vi "LEP_RV_PrepareBuild.vi"(5 "Rebuild":bool, 11 "error in (no error)":errorcluster) -> (0 "error string":string, 1 "Node ID List":i32[](array[numeric]), 2 "Active File Count":i32, 3 "TopLevelVI":path, 4 "UV License OK":bool, 6 "Config":T1={"Enable debugging"=FALSE, "Debug Options"=0, "Use stack variables"=FALSE, "Generate serial only"=FALSE, "Generate guard code"=TRUE, "Generate Integer Only"=TRUE, "Generate C Function Calls"=TRUE, "ExpressionFolding"=FALSE, "Constant Allocation"=0, "Constant Deallocation"=0, "Build Specification ID"="", "Preprocessor symbols (define)"="", "Compiler Flags"="", "Linker Flags"="", "Mode"=1, "Optimization"=2, "Optimize for time"=FALSE, "Enable cross-module optimization"=FALSE, "Include paths"=[], "Optimize heap size"=TRUE, "Use MicroLib"=FALSE, "Debug Mode"=2, "Enable profile information"=FALSE, "Host name"="board", "Use DHCP"=TRUE, "IP address"="0.0.0.0", "Subnet mask"="", "Gateway"="0.0.0.0", "Primary DNS"="0.0.0.0", "Secondary DNS"="0.0.0.0", "MAC in target memory"=TRUE, "MAC address"="", "Console output"=1, "Target serial port"=1} {"Constant Deallocation" items=["Out of Scope", "VI End", "Application End"]; "Constant Allocation" items=["First Use", "Containing Loop", "VI Initialization", "Application Initialization"]; "Target serial port" items=["0", "1", "2", "3"]; "Console output" items=["Processor status window", "Serial port"]; "Optimization" items=["Level 0 (-O0)", "Level 1 (-O1)", "Level 2 (-O2)", "Level 3 (-O3)"]; "Mode" items=["ARM-Mode", "Thumb-Mode"]; "Debug Options" items=["Use ULINK Debugger", "Use Simulator"]; "Debug Mode" items=["Instrumented (serial port)", "Instrumented (TCP/IP)", "Non-instrumented (JTAG/USB)"]}, 8 "Build Path":path, 10 "Target Name":string, 12 "Message List":string[][](array[string]), 13 "Error Indicator":bool[](array[boolean]), 14 "UV Project File":path, 15 "error out":errorcluster)   [LabVIEW 2011]
doc: "Loads project configuration information, creates the build folder, prepares the source files, builds, and links the embedded application."
uses:
  LEP_RV_Config.ctl
panel:
  out "Executable file":path
  in  "Build Path":path
  in  "Config":T1={"Enable debugging"=FALSE, "Debug Options"=0, "Use stack variables"=FALSE, "Generate serial only"=FALSE, "Generate guard code"=FALSE, "Generate Integer Only"=FALSE, "Generate C Function Calls"=TRUE, "ExpressionFolding"=TRUE, "Constant Allocation"=0, "Constant Deallocation"=0, "Build Specification ID"="", "Preprocessor symbols (define)"="", "Compiler Flags"="", "Linker Flags"="", "Mode"=1, "Optimization"=2, "Optimize for time"=FALSE, "Enable cross-module optimization"=FALSE, "Include paths"=[], "Optimize heap size"=TRUE, "Use MicroLib"=FALSE, "Debug Mode"=2, "Enable profile information"=FALSE, "Host name"="board", "Use DHCP"=TRUE, "IP address"="0.0.0.0", "Subnet mask"="", "Gateway"="0.0.0.0", "Primary DNS"="0.0.0.0", "Secondary DNS"="0.0.0.0", "MAC in target memory"=TRUE, "MAC address"="", "Console output"=1, "Target serial port"=1} {"Constant Deallocation" items=["Out of Scope", "VI End", "Application End"]; "Constant Allocation" items=["First Use", "Containing Loop", "VI Initialization", "Application Initialization"]; "Target serial port" items=["0", "1", "2", "3"]; "Console output" items=["Processor status window", "Serial port"]; "Optimization" items=["Level 0 (-O0)", "Level 1 (-O1)", "Level 2 (-O2)", "Level 3 (-O3)"]; "Mode" items=["ARM-Mode", "Thumb-Mode"]; "Debug Options" items=["Use ULINK Debugger", "Use Simulator"]; "Debug Mode" items=["Instrumented (serial port)", "Instrumented (TCP/IP)", "Non-instrumented (JTAG/USB)"]}
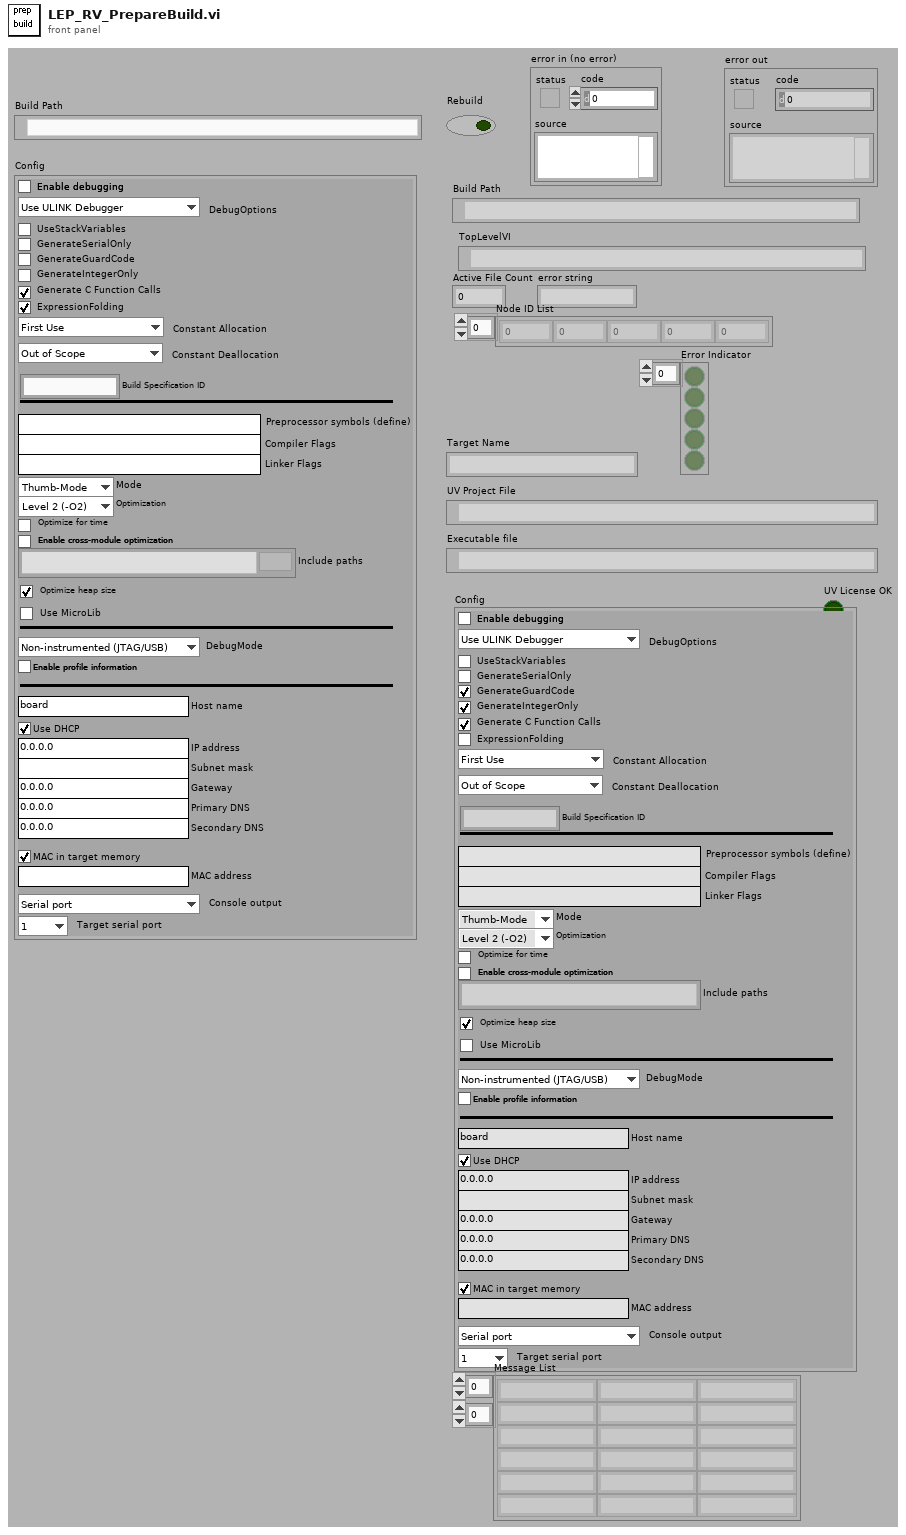
[diagram p1: front panel]
types:
  T1 = typedef "LEP_RV_Config.ctl" = cluster{"Enable debugging":bool, "Debug Options":u16, "Use stack variables":bool, "Generate serial only":bool, "Generate guard code":bool, "Generate Integer Only":bool, "Generate C Function Calls":bool, "ExpressionFolding":bool, "Constant Allocation":u16, "Constant Deallocation":u16, "Build Specification ID":string, "Preprocessor symbols (define)":string, "Compiler Flags":string, "Linker Flags":string, "Mode":u16, "Optimization":u16, "Optimize for time":bool, "Enable cross-module optimization":bool, "Include paths":path[], "Optimize heap size":bool, "Use MicroLib":bool, "Debug Mode":u16, "Enable profile information":bool, "Host name":string, "Use DHCP":bool, "IP address":string, "Subnet mask":string, "Gateway":string, "Primary DNS":string, "Secondary DNS":string, "MAC in target memory":bool, "MAC address":string, "Console output":u16, "Target serial port":u16}
  T2 = enum16{"NoErr", "TopLevelVIErr", "EmptyTopLevelVIPath", "CGenErr", "CpySuppFilesErr", "ProjectInfoErr", "NoTopLevelVIErr", "CreateBuildFolderErr", "EmptyBuildFolderErr", "LoadConfigErr", "BildToolsErr", "CompileErr", "LinkError", "DebugInfoErr", "NotFoundErr", "AccessErr", "ExecErr", "UnknownErr", "ISRErr"}
  T3 = enum16{"LoadProjectInfo", "LoadConfig", "SetupBuildFolder", "CopySupportFiles", "CGen", "CreateUVProject", "ConfigureUVproject", "BuildwithUV", "GenerateDebugDatabase", "ShowUserMessage", "Done", "Error"}
  T4 = enum16{"Normal", "Minimized", "Maximized", "Hidden", "Locked"}
  T5 = enum16{"NoErr", "TopLevelVIErr", "EmptyTopLevelVIPath", "CGenErr", "CpySuppFilesErr", "ProjectInfoErr", "NoTopLevelVIErr", "CreateBuildFolderErr", "EmptyBuildFolderErr", "LoadConfigErr", "BildToolsErr", "CompileErr", "LinkError", "DebugInfoErr", "NotFoundErr", "AccessErr", "ExecErr", "UnknownErr"}
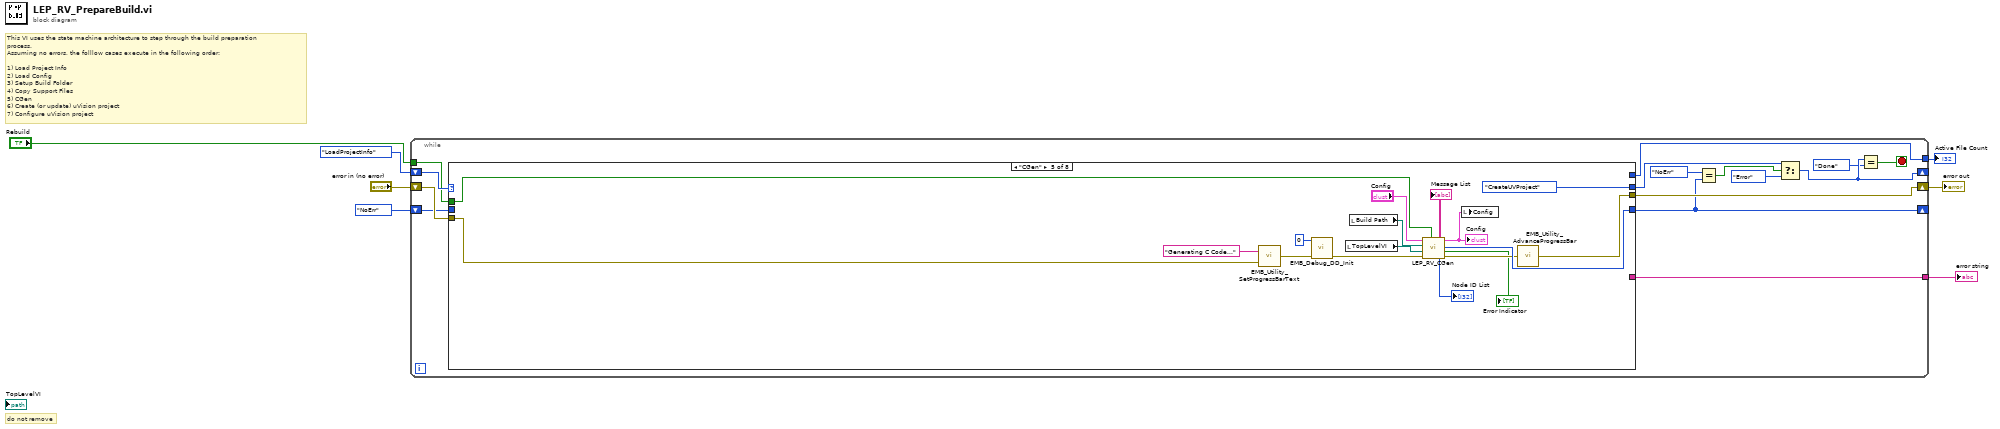
[diagram p0: block diagram]
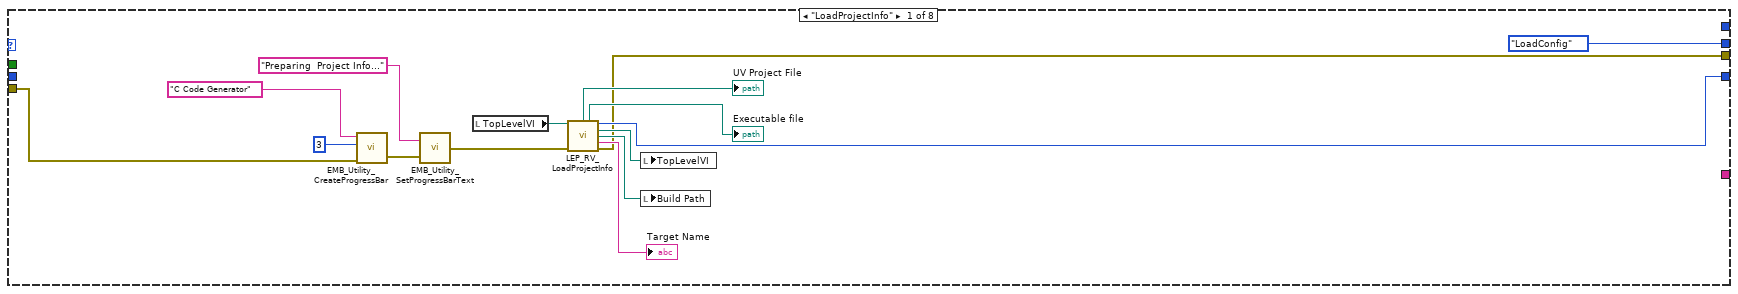
[diagram p2: hidden frame]
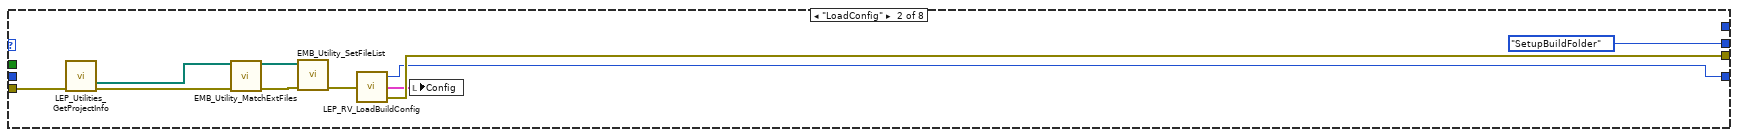
[diagram p3: hidden frame]
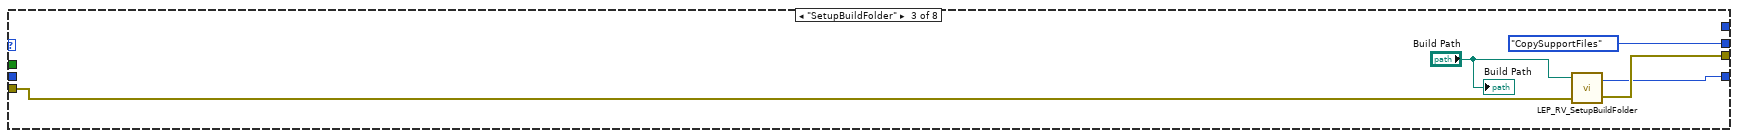
[diagram p4: hidden frame]
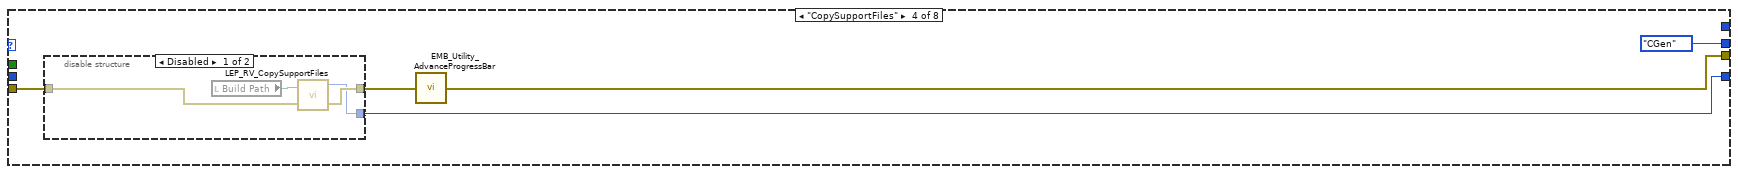
[diagram p5: hidden frame]
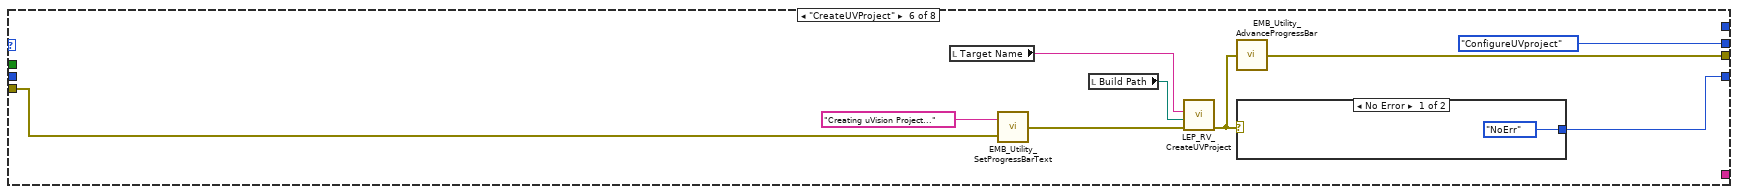
[diagram p7: hidden frame]
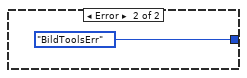
[diagram p8: hidden frame]
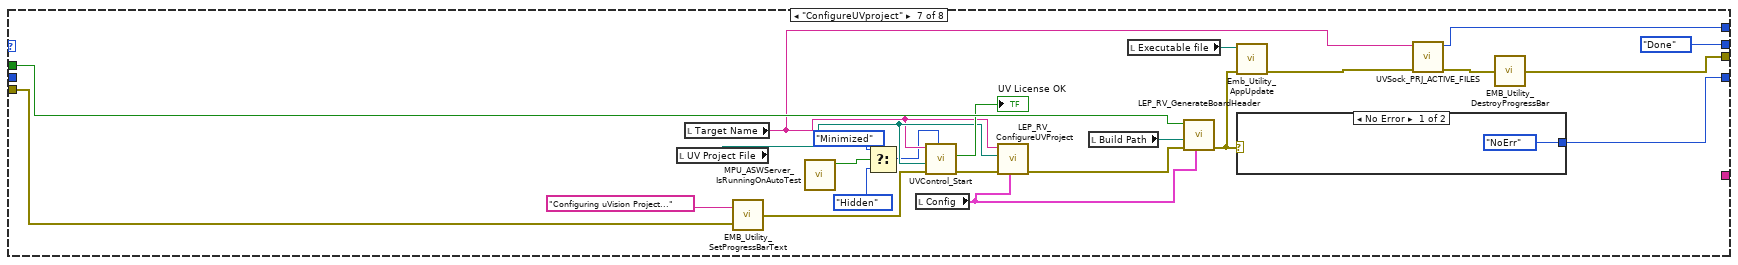
[diagram p9: hidden frame]
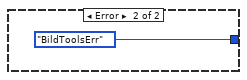
[diagram p10: hidden frame]
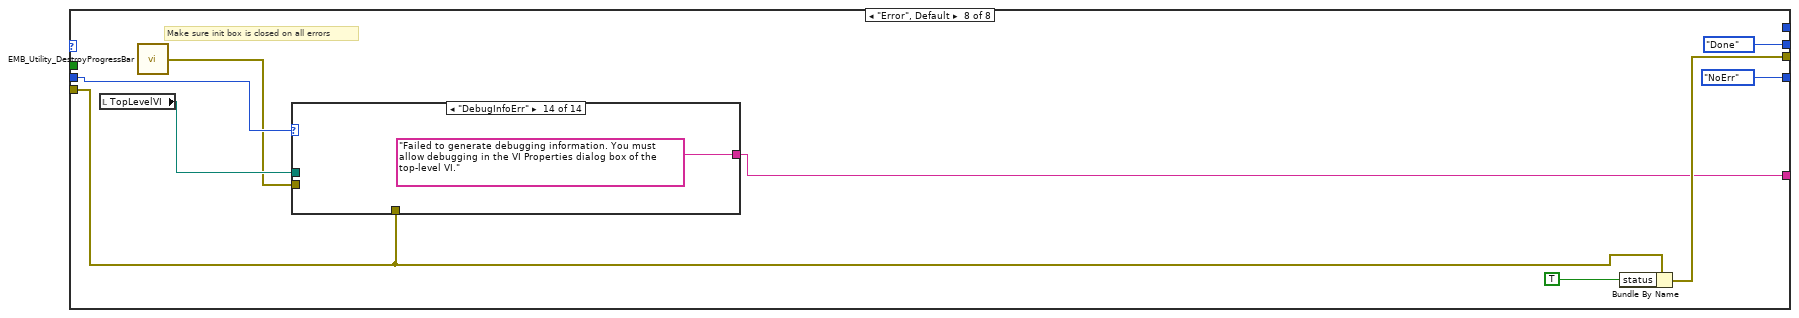
[diagram p11: hidden frame]
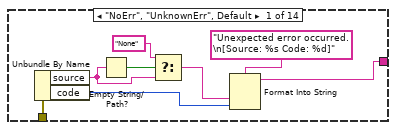
[diagram p12: hidden frame]
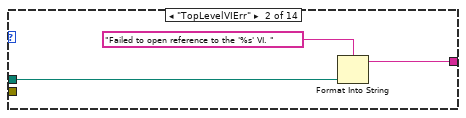
[diagram p13: hidden frame]
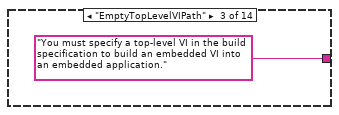
[diagram p14: hidden frame]
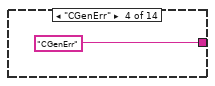
[diagram p15: hidden frame]
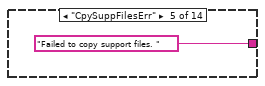
[diagram p16: hidden frame]
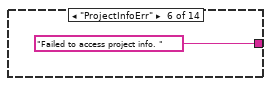
[diagram p17: hidden frame]
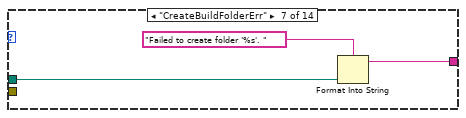
[diagram p18: hidden frame]
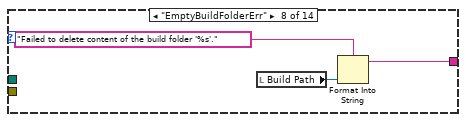
[diagram p19: hidden frame]
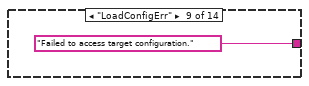
[diagram p20: hidden frame]
diagram:
  # "do not remove"
  # "This VI uses the state machine architecture to step through the build preparation process.\nAssuming no errors, the folllow cases execute in the following order:\n\n1) Load Project Info\n2) Load Config\n3) Setup Build Folder\n4) Copy Support Files\n5) CGen\n6) Create (or update) uVision project\n7) Configure uVision project"
  n1 = while {
    shift-right: [w20] -> w4
    shift-left: "error in (no error)" -> [w21]
    shift-right: [w15] -> _
    shift-left: T3."LoadProjectInfo" ("Phase") -> [w22]
    shift-right: [w13] -> _
    shift-left: T2."NoErr" ("Errors") -> [w19]
    tunnel: "Rebuild" -> [w11]
    tunnel: [w9] -> w2
    tunnel: [w8] -> w1
    stop <- w16 stop-if-true
    n2 = case shown="\"CGen\"" w22 {
      tunnel: w21 -> [w26 w40 w51 w57 w69 w83 w100 w116]
      tunnel: [w30 w47 w52 w53 w66 w80 w102 w119] -> w20
      tunnel: [w31 w46 w50 w56 w79 w87 w112 T2."NoErr" ("Errors")] -> w13
      tunnel: w19 -> [_ _ _ _ _ _ _ w122]
      tunnel: [T3."LoadConfig" ("Phase") T3."SetupBuildFolder" ("Phase") T3."CopySupportFiles" ("Phase") T3."CGen" ("Phase") T3."CreateUVProject" ("Phase") T3."ConfigureUVproject" ("Phase") T3."Done" ("Phase") T3."Done" ("Phase")] -> w17
      tunnel: w11 -> [_ _ _ _ w71 _ w108 _]
      tunnel: [_ _ _ _ _ _ w97 _] -> w9
      tunnel: [_ _ _ _ _ _ _ w117] -> w8
      frame "LoadProjectInfo" {
        n3 = call <vilib>:"EMB_Utility_CreateProgressBar.vi"("error in (no error)"=w26, "Steps"=u32 3, "Title"="C Code Generator") -> ("error out"=w24:errorcluster)  [unwired: 1 in, 1 out]
        n4 = call <vilib>:"EMB_Utility_SetProgressBarText.vi"("error in (no error)"=w24, "Step Text"="Preparing  Project Info..." ("Title")) -> ("error out"=w23:errorcluster)
        n5 = local read "TopLevelVI"() -> (w29:path)
        n6 = call "LEP_RV_LoadProjectInfo.vi"("TopLevelVIPath In"=w29, "error in (no error)"=w23) -> ("Project File"=→"UV Project File":path, "Executable File"=→"Executable file":path, "Status"=w31:T5, "TopLevelVIPath Out"=w37:path, "Build Path"=w34:path, "Target Name"=→"Target Name":string, "error out"=w30:errorcluster)  [unwired: 7 out]
        n7 = local write "TopLevelVI"(w37) -> ()
        n8 = local write "Build Path"(w34) -> ()
      }
      frame "LoadConfig" {
        n9 = call <vilib>:"LEP_Utilities_GetProjectInfo.vi"("error in"=w40) -> ("ExternalFiles"=w43:path[], "error out"=w41:errorcluster)  [unwired: 13 out]
        n10 = call <vilib>:"EMB_Utility_MatchExtFiles.vi"("ExternalFiles"=w43, "error in"=w41) -> ("MatchedFiles"=w44:path[], "error out"=w42:errorcluster)  [unwired: 1 in, 11 out]
        n11 = call <vilib>:"EMB_Utility_SetFileList.vi"("error in (no error)"=w42, "File List"=w44) -> ("error out"=w39:errorcluster)  [unwired: 9 out]
        n12 = call "LEP_RV_LoadBuildConfig.vi"("error in (no error)"=w39) -> ("Status"=w46:T5, "Config"=w45:T1, "error out"=w47:errorcluster)
        n13 = local write "Config"(w45) -> ()
      }
      frame "SetupBuildFolder" {
        n14 = call "LEP_RV_SetupBuildFolder.vi"("error in (no error)"=w51, "Build Path"="Build Path") -> ("error out"=w52:errorcluster, "Status"=w50:T5)  [unwired: 1 in]
        "Build Path" <- "Build Path"
      }
      frame "CopySupportFiles" {
        n15 = disable-structure shown="Disabled" {
          disable-tunnel: w57 -> [w61 w62]
          disable-tunnel: [w60 w62] -> w54
          disable-tunnel: [w59 _] -> w56
          frame Disabled {
            n16 = local read "Build Path"() -> (w58:path)
            n17 = call "LEP_RV_CopySupportFiles.vi"("error in (no error)"=w61, "Build Folder"=w58) -> ("error out"=w60:errorcluster, "Status"=w59:T5)
          }
          frame Enabled {
          }
        }
        n18 = call <vilib>:"EMB_Utility_AdvanceProgressBar.vi"("error in (no error)"=w54) -> ("error out"=w53:errorcluster)
      }
      frame "CGen" {
        n19 = call <vilib>:"EMB_Utility_SetProgressBarText.vi"("error in (no error)"=w69, "Step Text"="Generating C Code..." ("Title")) -> ("error out"=w68:errorcluster)
        n20 = call <vilib>:"EMB_Debug_DD_Init.vi"("error in (no error)"=w68, "target ID"=u32 0) -> ("error out"=w73:errorcluster)  [unwired: 9 out]
        n21 = local read "TopLevelVI"() -> (w78:path)
        n22 = local read "Build Path"() -> (w75:path)
        n23 = call "LEP_RV_CGen.vi"("Rebuild"=w71, "error in (no error)"=w73, "Top Level VI"=w78, "Destination Folder"=w75, "Configuration"="Config") -> ("error out"=w67:errorcluster, "Error Indicator"=→"Error Indicator":bool[], "Status"=w79:T2, "Configuration"=w72:T1, "Node ID List"=→"Node ID List":i32[], "Message List"=→"Message List":string[][])  [unwired: 1 out]
        "Config" <- w72
        n24 = local write "Config"(w72) -> ()
        n25 = call <vilib>:"EMB_Utility_AdvanceProgressBar.vi"("error in (no error)"=w67) -> ("error out"=w66:errorcluster)
      }
      frame "CreateUVProject" {
        n26 = local read "Target Name"() -> (w85:string)
        n27 = call <vilib>:"EMB_Utility_SetProgressBarText.vi"("error in (no error)"=w83, "Step Text"="Creating uVision Project..." ("Title")) -> ("error out"=w82:errorcluster)
        n28 = local read "Build Path"() -> (w86:path)
        n29 = call "LEP_RV_CreateUVProject.vi"("error in (no error)"=w82, "Build Path"=w86, "Target"=w85) -> ("error out"=w81:errorcluster)  [unwired: 8 out]
        n30 = call <vilib>:"EMB_Utility_AdvanceProgressBar.vi"("error in (no error)"=w81) -> ("error out"=w80:errorcluster)
        n31 = case shown="No Error" w81 {
          tunnel: [T2."NoErr" ("Errors") T2."BildToolsErr" ("Errors")] -> w87
          frame No Error {
          }
          frame Error {
          }
        }
      }
      frame "ConfigureUVproject" {
        n32 = local read "UV Project File"() -> (w106:path)
        n33 = local read "Target Name"() -> (w95:string)
        n34 = call <vilib>:"EMB_Utility_SetProgressBarText.vi"("error in (no error)"=w100, "Step Text"="Configuring uVision Project..." ("Title")) -> ("error out"=w99:errorcluster)
        n35 = call <vilib>:"MPU_ASWServer_IsRunningOnAutoTest.vi"() -> ("running in autotest?"=w93:bool)  [unwired: 1 in, 10 out]
        n36 = Select(t=T4."Minimized", s=w93, f=T4."Hidden" ("Mode")) -> (s? t:f=w91:T4)
        n37 = local read "Config"() -> (w110:T1)
        n38 = call "UVControl_Start.vi"("Mode"=w91, "error in (no error)"=w99, "Project File"=w106, "Target"=w95) -> ("error out"=w113:errorcluster, "License OK"=→"UV License OK":bool)  [unwired: 1 in, 5 out]
        n39 = call "LEP_RV_ConfigureUVProject.vi"("Config"=w110, "error in (no error)"=w113, "uVision Project"=w106, "Target"=w95) -> ("error out"=w111:errorcluster)  [unwired: 1 in, 6 out]
        n40 = local read "Build Path"() -> (w109:path)
        n41 = local read "Executable file"() -> (w104:path)
        n42 = call "LEP_RV_GenerateBoardHeader.vi"("Config"=w110, "error in (no error)"=w111, "Build Path"=w109, "Rebuild"=w108) -> ("error out"=w103:errorcluster)  [unwired: 7 out]
        n43 = call <vilib>:"Emb_Utility_AppUpdate.vi"("error in (no error)"=w103, "Path"=w104) -> ("error out"=w96:errorcluster)  [unwired: 9 out]
        n44 = case shown="No Error" w103 {
          tunnel: [T2."NoErr" ("Errors") T2."BildToolsErr" ("Errors")] -> w112
          frame No Error {
          }
          frame Error {
          }
        }
        n45 = call "UVSock_PRJ_ACTIVE_FILES.vi"("error in (no error)"=w96, "Target"=w95) -> ("error out"=w98:errorcluster, "Active File Count"=w97:i32)  [unwired: 4 out]
        n46 = call <vilib>:"EMB_Utility_DestroyProgressBar.vi"("error in (no error)"=w98) -> ("error out"=w102:errorcluster)
      }
      frame "Error", Default {
        # "Make sure init box is closed on all errors"
        n47 = local read "TopLevelVI"() -> (w124:path)
        n48 = call <vilib>:"EMB_Utility_DestroyProgressBar.vi"() -> ("error out"=w120:errorcluster)  [unwired: 1 in]
        n49 = case shown="\"DebugInfoErr\"" w122 {
          tunnel: [w129 w133 "You must specify a top-level VI in the build specification to build an embedded VI into an embedded application." "CGenErr" "Failed to copy support files. " "Failed to access project info. " w140 w145 "Failed to access target configuration." "Compiler error occurred." "Linker error occurred." "Unknown error occurred." "Failed to generate C code.  Ensure that the project's interrupts are properly configured." "Failed to generate debugging information. You must allow debugging in the VI Properties dialog box of the top-level VI."] -> w117
          tunnel: w124 -> [_ w135 _ _ _ _ w141 _ _ _ _ _ _ _]
          tunnel: w120 -> [_ _ _ _ _ _ _ _ _ _ _ _ _ _]
          tunnel: w116 -> [w132 _ _ _ _ _ _ _ _ _ _ _ _ _]
          frame "NoErr", "UnknownErr", Default {
            n50 = Unbundle By Name(w132) -> ("source"=w126:string, "code"=w130:i32)
            n51 = Empty String/Path?(string/path=w126) -> (empty?=w128:bool)
            n52 = Select(t="None", s=w128, f=w126) -> (s? t:f=w125:string)
            n53 = Format Into String(format string="Unexpected error occurred.\n[Source: %s Code: %d]", w125, w130) -> (resulting string=w129:string)  [unwired: 2 in, 1 out]
          }
          frame "TopLevelVIErr" {
            n54 = Format Into String(format string="Failed to open reference to the '%s' VI. ", w135) -> (resulting string=w133:string)  [unwired: 2 in, 1 out]
          }
          frame "EmptyTopLevelVIPath" {
          }
          frame "CGenErr" {
          }
          frame "CpySuppFilesErr" {
          }
          frame "ProjectInfoErr" {
          }
          frame "CreateBuildFolderErr" {
            n55 = Format Into String(format string="Failed to create folder '%s'. ", w141) -> (resulting string=w140:string)  [unwired: 2 in, 1 out]
          }
          frame "EmptyBuildFolderErr" {
            n56 = local read "Build Path"() -> (w143:path)
            n57 = Format Into String(format string="Failed to delete content of the build folder '%s'.", w143) -> (resulting string=w145:string)  [unwired: 2 in, 1 out]
          }
          frame "LoadConfigErr" {
          }
          frame "CompileErr" {
          }
          frame "LinkError" {
          }
          frame "ExecErr" {
          }
          frame "ISRErr" {
          }
          frame "DebugInfoErr" {
          }
        }
        n58 = Bundle By Name(cluster=w116, "status"=TRUE) -> (w119:errorcluster)
      }
    }
    n59 = Equal?(x=T2."NoErr" ("Errors"), y=w13) -> (x = y?=w18:bool)
    n60 = Select(t=w17, s=w18, f=T3."Error" ("Phase")) -> (s? t:f=w15:T3)
    n61 = Equal?(x=w15, y=T3."Done" ("Phase")) -> (x = y?=w16:bool)
  }
  "error out" <- w4
  "Active File Count" <- w2
  "error string" <- w1
